vi "BME_DG_SetTriggerParameters.vi"(8 "error in (no error)":errorcluster, 10 "Trigger Settings":T1={"InputTerminated?"=FALSE, "InternalClockPeriode(µs)"=1000000.0, "TriggerLevel"=1.25, "PresetValue"=0, "DivideBy"=1, "Clock Source"=1, "Gate Divider"=1, "PositiveGate?"=TRUE, "InternalTrigger?"=FALSE, "InternalArm?"=FALSE, "SWTrigger?"=FALSE, "RisingEdge?"=FALSE, "StopOnPreset?"=FALSE, "ResetWhenDone?"=TRUE, "TriggerEnabled?"=TRUE} {"Gate Divider" min=1 max=1000000; "Clock Source" items=["Internal Oscillator"=1, "External Trigger"=2, "Trigger & Oscillator"=3]; "InternalClockPeriode(µs)" format="%#_11g"}, 11 "DG_NumberM":i32) -> (0 "error out":errorcluster, 3 "return code":i32)   [LabVIEW 2009]
uses:
  BME_DG_TriggerSettings.ctl
  BME DLL/DelayGenerator.dll
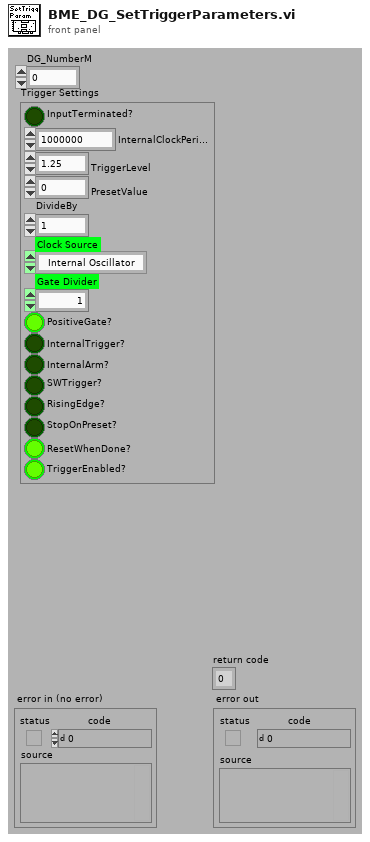
[diagram p1: front panel]
types:
  T1 = typedef "BME_DG_TriggerSettings.ctl" = cluster{"InputTerminated?":bool, "InternalClockPeriode(µs)":dbl, "TriggerLevel":dbl, "PresetValue":i32, "DivideBy":i32, "Clock Source":u32, "Gate Divider":i32, "PositiveGate?":bool, "InternalTrigger?":bool, "InternalArm?":bool, "SWTrigger?":bool, "RisingEdge?":bool, "StopOnPreset?":bool, "ResetWhenDone?":bool, "TriggerEnabled?":bool}
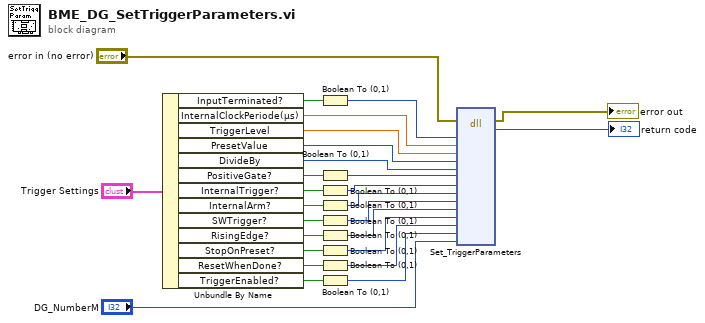
[diagram p0: block diagram]
diagram:
  n1 = Unbundle By Name("Trigger Settings") -> ("InputTerminated?"=w22:bool, "InternalClockPeriode(µs)"=w21:dbl, "TriggerLevel"=w20:dbl, "PresetValue"=w19:i32, "DivideBy"=w18:i32, "PositiveGate?"=w17:bool, "InternalTrigger?"=w15:bool, "InternalArm?"=w14:bool, "SWTrigger?"=w12:bool, "RisingEdge?"=w10:bool, "StopOnPreset?"=w8:bool, "ResetWhenDone?"=w6:bool, "TriggerEnabled?"=w3:bool)
  n2 = Boolean To (0,1)(Boolean=w22) -> (0, 1=w24:i16)
  n3 = Boolean To (0,1)(Boolean=w17) -> (0, 1=w16:i16)
  n4 = Boolean To (0,1)(Boolean=w15) -> (0, 1=w26:i16)
  n5 = Boolean To (0,1)(Boolean=w14) -> (0, 1=w13:i16)
  n6 = Boolean To (0,1)(Boolean=w12) -> (0, 1=w11:i16)
  n7 = Boolean To (0,1)(Boolean=w10) -> (0, 1=w9:i16)
  n8 = Boolean To (0,1)(Boolean=w8) -> (0, 1=w7:i16)
  n9 = Boolean To (0,1)(Boolean=w6) -> (0, 1=w5:i16)
  n10 = Boolean To (0,1)(Boolean=w3) -> (0, 1=w4:i16)
  n11 = dll-call lib="C:/Dokumente und Einstellungen/User/Desktop/POLARIS BME DG/BME DLL/DelayGenerator.dll" fn="Set_TriggerParameters"(error in="error in (no error)", "TriggerTerminate"=w24, "InternalClock"=w21, "TriggerLevel"=w20, "PresetValue"=w19, "GateDivider"=w18, "PositiveGate"=w16, "InternalTrigger"=w26, "InternalArm"=w13, "SoftwareTrigger"=w11, "RisingEdge"=w9, "StopOnPreset"=w7, "ResetWhenDone"=w5, "TriggerEnable"=w4, "DG_Number"="DG_NumberM") -> (error out=→"error out":errorcluster, →"return code":i32)  [unwired: 16 in, 1 out]
